vi "stiltLock.vi"(0 "Powered Lock SolenoidDevRef":T1={"DevStatus"={"status"=FALSE, "code"=0, "source"=""}, "Pneumatics Control Module"=0, "Forward Solenoid Channel"=enum."Invalid", "Reverse Solenoid Channel"=enum."Invalid"}, 1 "Skid Lock SolenoidDevRef":T1={"DevStatus"={"status"=FALSE, "code"=0, "source"=""}, "Pneumatics Control Module"=0, "Forward Solenoid Channel"=enum."Invalid", "Reverse Solenoid Channel"=enum."Invalid"}, 2 "Lock State":T3(ring)) -> ()   [LabVIEW 2018]
uses:
  <vilib>/Rock Robotics/WPI/Solenoid/WPI_SolenoidDevRef.ctl
  <vilib>/Rock Robotics/WPI/Solenoid/WPI_SolenoidChannel.ctl
  <vilib>/Rock Robotics/WPI/Solenoid/WPI_SolenoidValue.ctl
  <userlib>/836-Library/System/TDMS_V2/Support/TDMS_DevRef.ctl
  <userlib>/836-Library/System/TDMS_V2/Support/Logging_Settings.ctl
  <userlib>/836-Library/System/TDMS_V2/Support/Group_FIFO_Config.ctl
  <userlib>/836-Library/System/TDMS_V2/Support/Channel_FIFO_Config.ctl
  <vilib>/Rock Robotics/WPI/Solenoid/WPI_SolenoidSetEnum.vi
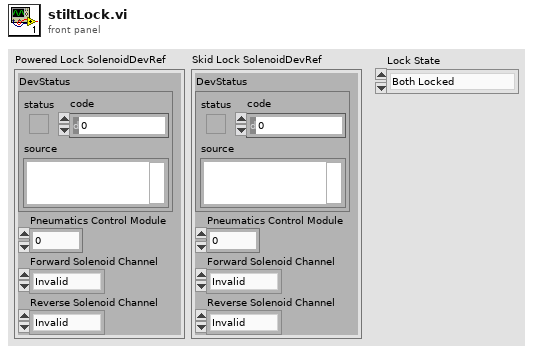
[diagram p1: front panel]
types:
  T1 = typedef "WPI_SolenoidDevRef.ctl" = cluster{"DevStatus":errorcluster, "Pneumatics Control Module":u8, "Forward Solenoid Channel":T2, "Reverse Solenoid Channel":T2}
  T2 = typedef "WPI_SolenoidChannel.ctl" = enum8{"Solenoid 0", "Solenoid 1", "Solenoid 2", "Solenoid 3", "Solenoid 4", "Solenoid 5", "Solenoid 6", "Solenoid 7", "Invalid"}
  T3 = enum16{"Both Locked", "Skid Unlock/Powered Locked", "Skid Locked/Powered Unlocked", "Both Unlocked"}
  T4 = typedef "TDMS_DevRef.ctl" = cluster{"Name":string, "File Ref":refnum<k34>, "Start Time":timestamp, "Logging Settings":T5, "Group FIFO Config":T6[], "Data To Write":refnum<data-value>, "semaphore":T8, "Ref Time Reset":refnum<k4>}
  T5 = typedef "Logging_Settings.ctl" = cluster{"Data Grab Period":dbl, "File Write Period":dbl, "Max Stored Size":dbl, "Burst Size":dbl}
  T6 = typedef "Group_FIFO_Config.ctl" = cluster{"Group":string, "Channels":T7[], "Channel Names":string[]}
  T7 = typedef "Channel_FIFO_Config.ctl" = cluster{"Channel":string, "FIFO":refnum<k33>}
  T8 = typedef "Semaphore RefNum" = refnum<k1>
  T9 = typedef "WPI_SolenoidValue.ctl" = enum16{"Off", "On", "Forward", "Reverse"}
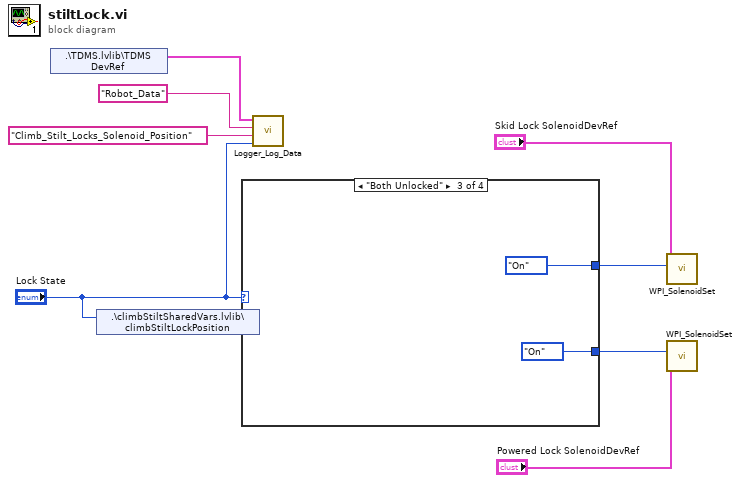
[diagram p0: block diagram]
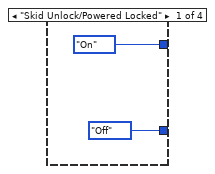
[diagram p2: hidden frame]
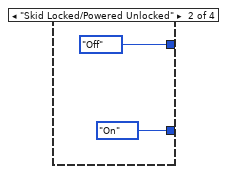
[diagram p3: hidden frame]
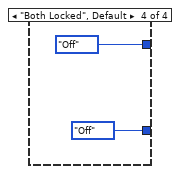
[diagram p4: hidden frame]
diagram:
  n1 = shared-variable ".\\TDMS.lvlib\\TDMS DevRef"() -> (w2:T4)  [unwired: 1 in, 1 out]
  n2 = shared-variable ".\\climbStiltSharedVars.lvlib\\climbStiltLockPosition"("Lock State") -> ()  [unwired: 1 in, 1 out]
  n3 = case shown="\"Both Unlocked\"" "Lock State" {
    tunnel: [WPI_SolenoidValue."Off" ("Value") WPI_SolenoidValue."On" ("Value") WPI_SolenoidValue."On" ("Value") WPI_SolenoidValue."Off" ("Value")] -> w8
    tunnel: [WPI_SolenoidValue."On" ("Value") WPI_SolenoidValue."Off" ("Value") WPI_SolenoidValue."On" ("Value") WPI_SolenoidValue."Off" ("Value")] -> w7
    frame "Skid Unlock/Powered Locked" {
    }
    frame "Skid Locked/Powered Unlocked" {
    }
    frame "Both Unlocked" {
    }
    frame "Both Locked", Default {
    }
  }
  n4 = call <userlib>:"Logger_Log_Data.vi"("Data"="Lock State", "Channel"="Climb_Stilt_Locks_Solenoid_Position", "Group"="Robot_Data", "TDMS DevRef"=w2) -> ()  [unwired: 7 in, 1 out]
  n5 = call-poly <vilib>:"WPI_SolenoidSet.vi"("Value"=w7, "SolenoidDevRef"="Skid Lock SolenoidDevRef") -> ()  [unwired: 8 in, 2 out]
  n6 = call-poly <vilib>:"WPI_SolenoidSet.vi"("Value"=w8, "SolenoidDevRef"="Powered Lock SolenoidDevRef") -> ()  [unwired: 8 in, 2 out]
